vi "RT Host Interleaving.vi"() -> ()   [LabVIEW 2012]
uses:
  <vilib>/rvi/interface/nirviOpenFPGA/nirviOpenFPGA.xnode
  <vilib>/rvi/interface/nirviCloseFPGA/nirviCloseFPGA.xnode
  <vilib>/rvi/interface/nirviMethod/nirviMethod.xnode
  <vilib>/rvi/interface/nirviReadWriteControl/nirviReadWriteControl.xnode
  FPGA Interleaving.vi
  <vilib>/rvi/errors/niLvFpgaMergeErrorWithErrorCode.vi
  <vilib>/rvi/errors/niLvFpgaAdjustHostInterfaceError.vi
  NiFpgaLv.dll
  <vilib>/Utility/error.llb/Error Cluster From Error Code.vi
  <vilib>/FPGAPlugInAG/cRIO-9074/niLvFpga_ReadFifo_cRIO-9074.vi
  <vilib>/FPGAPlugInAG/cRIO-9074/niLvFpga_Close_cRIO-9074.vi
panel:
  out "error out":errorcluster
  out "Overflow Count":u32
  in  "stop":bool
  in  "Samples per Channel":u32=1000
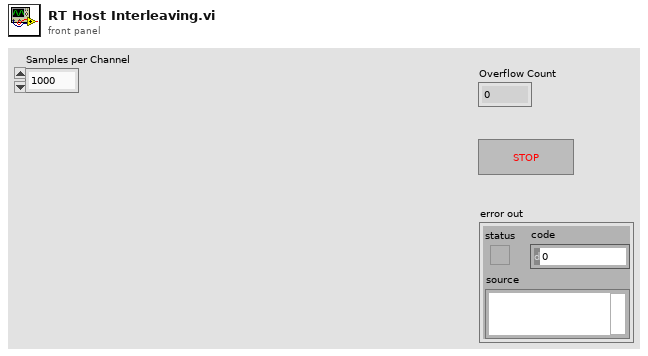
[diagram p1: front panel]
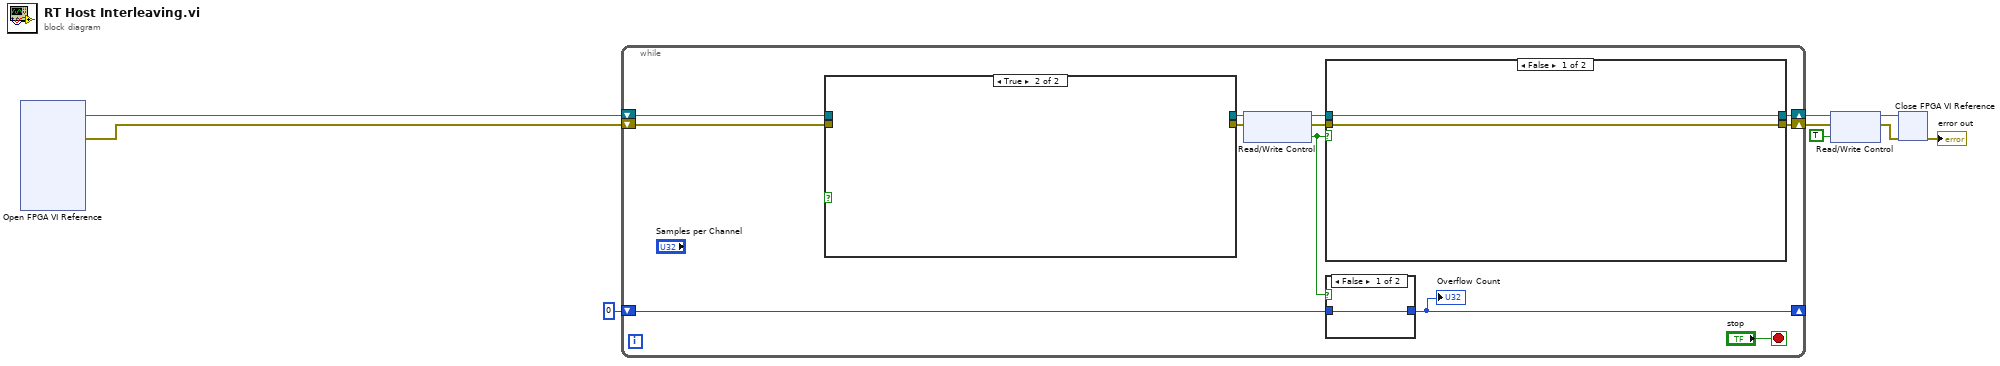
[diagram p0: block diagram]
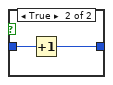
[diagram p2: hidden frame]
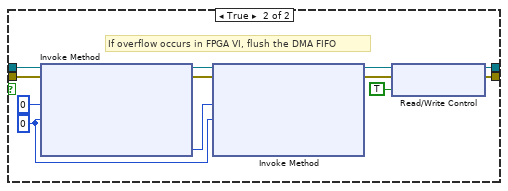
[diagram p4: hidden frame]
diagram:
  n1 = xnode "Open FPGA VI Reference"() -> ("FPGA VI Reference Out"=w1:refnum<k20>, "error out"=w2:errorcluster)  [unwired: 2 in]
  n2 = while {
    shift-right: [w19] -> w9
    shift-left: w1 -> [w11]
    shift-right: [w16] -> w5
    shift-left: w2 -> [w10]
    shift-right: [w13] -> _
    shift-left: u32 0 -> [w14]
    stop <- "stop" stop-if-true
    n3 = case shown="True" {
      selector: _ -> [_ _]
      tunnel: w11 -> [w26 _]
      tunnel: w10 -> [w25 _]
      tunnel: [w26 _] -> w18
      tunnel: [w25 _] -> w17
      frame False {
      }
      frame True {
      }
    }
    n4 = xnode "Read/Write Control"("FPGA VI Reference In"=w18, "error in"=w17) -> ("FPGA VI Reference Out"=w21:refnum<k20>, "error out"=w20:errorcluster, "Overflow?"=w12:bool)
    n5 = case shown="False" w12 {
      tunnel: w21 -> [w28 w40]
      tunnel: w20 -> [w27 w39]
      tunnel: [w28 w35] -> w19
      tunnel: [w27 w34] -> w16
      frame False {
      }
      frame True {
        w31 = 0 ("Timeout (ms)")
        # "If overflow occurs in FPGA VI, flush the DMA FIFO"
        n6 = xnode "Invoke Method"("FPGA VI Reference In"=w40, "error in"=w39, "Number of Elements"=u32 0, "Timeout (ms)"=w31) -> ("FPGA VI Reference Out"=w38:refnum<k20>, "error out"=w37:errorcluster, "Elements Remaining"=w32:u32)  [unwired: 1 out]
        n7 = xnode "Invoke Method"("FPGA VI Reference In"=w38, "error in"=w37, "Number of Elements"=w32, "Timeout (ms)"=w31) -> ("FPGA VI Reference Out"=w30:refnum<k20>, "error out"=w29:errorcluster)  [unwired: 2 out]
        n8 = xnode "Read/Write Control"("FPGA VI Reference In"=w30, "error in"=w29, "DMA Cleared?"=TRUE ("Reset")) -> ("FPGA VI Reference Out"=w35:refnum<k20>, "error out"=w34:errorcluster)
      }
    }
    n9 = case shown="False" w12 {
      tunnel: w14 -> [w22 w24]
      tunnel: [w22 w23] -> w13
      frame False {
      }
      frame True {
        n10 = Increment(x=w24) -> (x+1=w23:u32)
      }
    }
    "Overflow Count" <- w13
  }
  n11 = xnode "Read/Write Control"("FPGA VI Reference In"=w9, "error in"=w5, "stop"=TRUE) -> ("FPGA VI Reference Out"=w8:refnum<k20>, "error out"=w7:errorcluster)
  n12 = xnode "Close FPGA VI Reference"("FPGA VI Reference In"=w8, "error in"=w7) -> ("error out"=→"error out":errorcluster)
